vi "Do.vi"(8 "error in":errorcluster, 10 "Actor in":refnum<class "Actor.lvclass">, 11 "Update TEC PID":refnum<class "Update TEC PID.lvclass">) -> (0 "error out":errorcluster, 2 "Actor out":refnum<class "Actor.lvclass">)   [LabVIEW 2015, in "Generic TEC.lvlib" / "Update TEC PID.lvclass"]
doc: "(<B>Filename</B>: Actor Framework.lvlib:Message.lvclass:Do.vi)\n\nDefines what a message does when it is received by an actor. Generally, a message instructs an actor to invoke one of its methods. By default, this method does nothing. A child class must override it to define behavior. Create a child class by using the Actor Framework Message Maker dialog box."
uses:
  Update TEC PID.lvclass
  <vilib>/ActorFramework/Actor/Actor.lvclass
  TEC.lvclass
  <vilib>/MSR Consulting, LLC/Devices/DAQ Device/Device/Device.lvclass
  <vilib>/MSR Consulting, LLC/Devices/DAQ Device/Device/Device.lvclass/Device.ctl
  <vilib>/MSR Consulting, LLC/General Reuse/SuperActor/SuperActor.lvclass/SuperActor.ctl
  Update TEC PID.lvclass/Update TEC PID.ctl
  <vilib>/MSR Consulting, LLC/Devices/DAQ Device/Device/Read Configurable Device.vi
  <vilib>/MSR Consulting, LLC/General Reuse/SuperActor/Read ID.vi
  <vilib>/MSR Consulting, LLC/General Reuse/SuperActor/Read Log Session.vi
  <vilib>/MSR Consulting, LLC/General Reuse/SuperActor/Read CVT Session.vi
  <vilib>/MSR Consulting, LLC/Devices/Configurable Device/Configurable Device.lvclass
  <vilib>/MSR Consulting, LLC/General Reuse/Session APIs/_Session Fwk/Session - Root.lvclass
  <vilib>/MSR Consulting, LLC/General Reuse/Session APIs/CVT/CVT.lvclass
  <vilib>/MSR Consulting, LLC/General Reuse/Session APIs/Session Log/System Log.lvclass
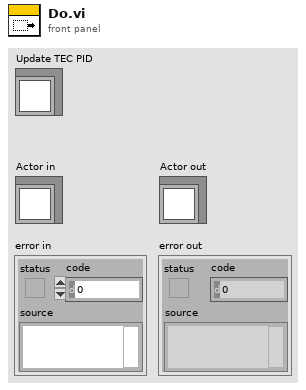
[diagram p1: front panel]
types:
  T1 = typedef "Session - Root.lvclass/Session Handle.ctl" = refnum<data-value>
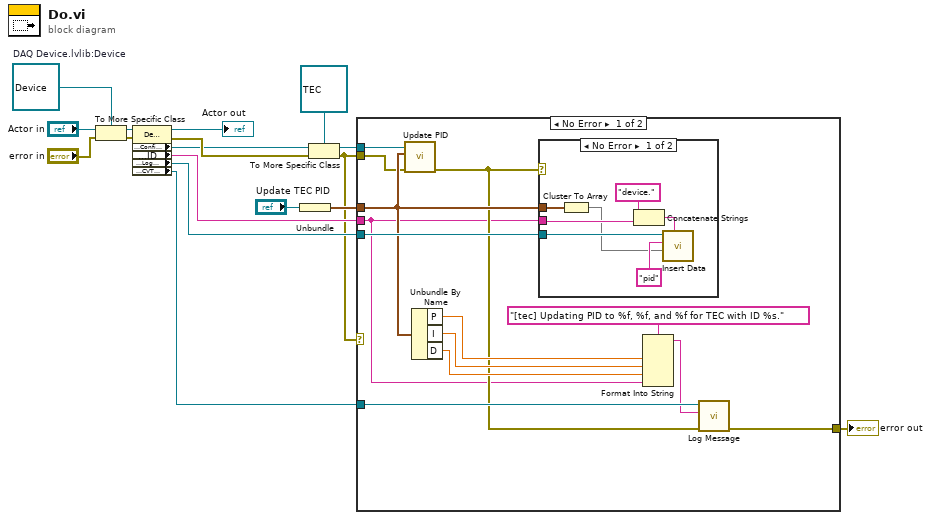
[diagram p0: block diagram]
diagram:
  w1 = refnum<class "Device.lvclass"> refnum  # DAQ Device.lvlib:Device
  n1 = To More Specific Class(target class=w1, reference="Actor in", error in="error in") -> (specific class reference=w16:refnum<class "Device.lvclass">, error out=w13:errorcluster)
  n2 = property class="Device"(reference=w16, error in=w13) -> (reference out=→"Actor out":refnum<class "Device.lvclass">, error out=w15:errorcluster, "Accessors:Configurable Device"=w2:refnum<class "Configurable Device.lvclass">, "Accessors:ID"=w4:string, "Accessors:Log Session"=w11:T1, "Accessors:CVT Session"=w10:T1)
  n3 = Unbundle("Update TEC PID") -> (w5:cluster{"P":dbl, "I":dbl, "D":dbl})
  n4 = To More Specific Class(target class=refnum<class "TEC.lvclass"> refnum ("Generic TEC.lvlib:TEC"), reference=w2, error in=w15) -> (specific class reference=w6:refnum<class "TEC.lvclass">, error out=w3:errorcluster)
  n5 = case shown="No Error" w3 {
    tunnel: w11 -> [w30 _]
    tunnel: w10 -> [w29 _]
    tunnel: [w23 _] -> w9
    tunnel: w6 -> [w22 _]
    tunnel: w5 -> [w21 _]
    tunnel: w3 -> [w20 _]
    tunnel: w4 -> [w18 _]
    frame No Error {
      n6 = call-dynamic "Update PID.vi"("error in (no error)"=w20, "ctl"=w21, "TEC in"=w22) -> ("error out"=w19:errorcluster)  [unwired: 7 in, 1 out]
      n7 = Unbundle By Name(w21) -> ("P"=w27:dbl, "I"=w26:dbl, "D"=w25:dbl)
      n8 = case shown="No Error" w19 {
        tunnel: w30 -> [w34 _]
        tunnel: w18 -> [w35 _]
        tunnel: w21 -> [w32 _]
        frame No Error {
          n9 = Cluster To Array(cluster=w32) -> (array=w31:dbl[])
          n10 = Concatenate Strings("device." ("string"), w35) -> (w33:string)
          n11 = call <vilib>:"Insert Data.vi"("Group"=w33, "Data"=w31, "tag"="pid", "CVT Session In"=w34) -> ()  [unwired: 6 in, 2 out]
        }
        frame Error {
        }
      }
      n12 = Format Into String(format string="[tec] Updating PID to %f, %f, and %f for TEC with ID %s.", w27, w26, w25, w18) -> (resulting string=w24:string)  [unwired: 2 in, 1 out]
      n13 = call <vilib>:"Log Message.vi"("error in"=w19, "MSG In"=w24, "session in"=w29) -> ("error out"=w23:errorcluster)  [unwired: 7 in, 1 out]
    }
    frame Error {
      # "Went to wrong device - die silently..."
    }
  }
  "error out" <- w9
